vi "InitializeFromExample.vi"(8 "error in (no error)":errorcluster, 9 "StartingCameraFrame":i32, 10 "StimulusObjectIndex":i32, 11 "Stimulus in":refnum<class "StimulusObject.lvclass">) -> (0 "error out":errorcluster, 3 "Stimulus out":refnum<class "StimulusObject.lvclass">)   [LabVIEW 2019, in "StimulusObject.lvclass"]
uses:
  StimulusObject.lvclass
  StimulusObject.lvclass/StimulusObject.ctl
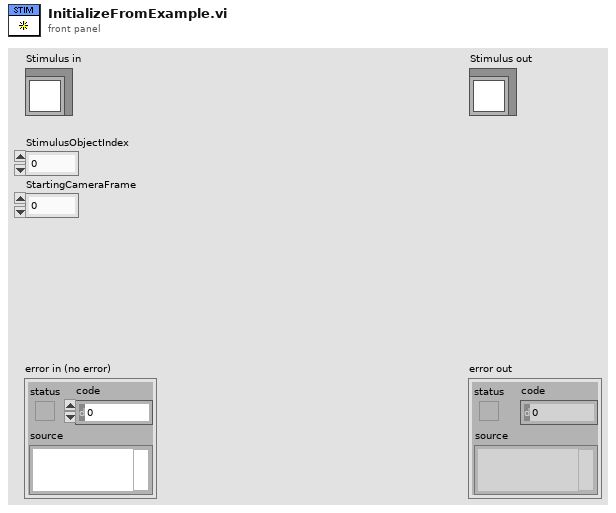
[diagram p1: front panel]
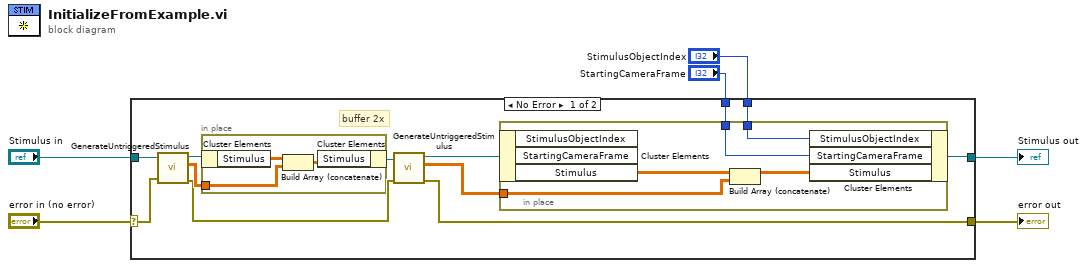
[diagram p0: block diagram]
diagram:
  n1 = case shown="No Error" "error in (no error)" {
    selector: "error in (no error)" -> [w17 w28]
    tunnel: [w18 w28] -> w5
    tunnel: [w14 w27] -> w3
    tunnel: "Stimulus in" -> [w16 w27]
    tunnel: "StartingCameraFrame" -> [w9 _]
    tunnel: "StimulusObjectIndex" -> [w8 _]
    frame No Error {
      # "buffer 2x"
      n2 = call-dynamic "GenerateUntriggeredStimulus.vi"("error in (no error)"=w17, "StimulusObject in"=w16) -> ("error out"=w7:errorcluster, "UntriggeredStimulusOut"=w10:sgl[][], "StimulusObject out"=w12:refnum<class "StimulusObject.lvclass">)  [unwired: 7 in]
      n3 = in-place {
        in-place-border: w10 -> [w19]
        n4 = in-place-cluster #1(w12) -> ("Stimulus"=w21:sgl[][])
        n5 = Build Array (concatenate)(w21, w19) -> (w20:sgl[][])
        n6 = in-place-cluster #1("Stimulus"=w20) -> (w11:refnum<class "StimulusObject.lvclass">)
      }
      n7 = call-dynamic "GenerateUntriggeredStimulus.vi"("error in (no error)"=w7, "StimulusObject in"=w11) -> ("error out"=w18:errorcluster, "UntriggeredStimulusOut"=w13:sgl[][], "StimulusObject out"=w15:refnum<class "StimulusObject.lvclass">)  [unwired: 7 in]
      n8 = in-place {
        in-place-border: w13 -> [w24]
        in-place-border: w9 -> [w23]
        in-place-border: w8 -> [w22]
        n9 = in-place-cluster #2(w15) -> ("Stimulus"=w26:sgl[][])  [unwired: 2 out]
        n10 = Build Array (concatenate)(w26, w24) -> (w25:sgl[][])
        n11 = in-place-cluster #2("StimulusObjectIndex"=w22, "StartingCameraFrame"=w23, "Stimulus"=w25) -> (w14:refnum<class "StimulusObject.lvclass">)
      }
    }
    frame Error {
    }
  }
  "error out" <- w5
  "Stimulus out" <- w3
